vi "BarIncreaserPractice.vi"() -> ()   [LabVIEW 2014]
panel:
  in  "stop":bool
  out "Slide":u8(slide) scale=0.0..100.0
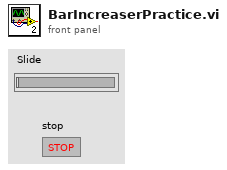
[diagram p1: front panel]
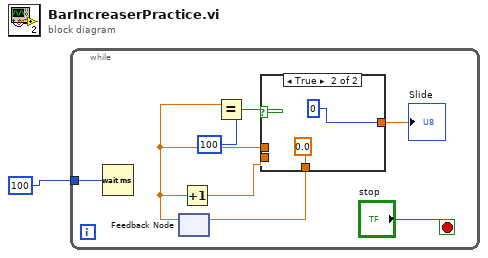
[diagram p0: block diagram]
diagram:
  n1 = while {
    tunnel: 100 -> [w8]
    stop <- "stop" stop-if-true
    n2 = Wait (ms)(milliseconds to wait=w8) -> ()  [unwired: 1 out]
    n3 = feedback #1() -> (w4:dbl)  [unwired: 1 in]
    n4 = Increment(x=w4) -> (x+1=w3:dbl)
    n5 = Equal?(x=w4, y=100) -> (x = y?=w6:bool)
    n6 = case shown="True" w6 {
      tunnel: [w11 0] -> w5
      tunnel: w4 -> [w11 _]
      tunnel: w3 -> [w10 _]
      tunnel: [w10 0.0] -> w2
      frame False {
      }
      frame True {
      }
    }
    "Slide" <- w5
    n7 = feedback-in #1(w2) -> ()
  }
